vi "Graph Data.vi"(8 "error in (no error)":errorcluster, 10 "signal out":waveform(dbl), 11 "GUI_Graph in":refnum<class "GUI_Graph.lvclass">) -> (0 "error out":errorcluster, 3 "GUI_Graph out":refnum<class "GUI_Graph.lvclass">)   [LabVIEW 2020, in "GUI_Graph.lvlib" / "GUI_Graph.lvclass"]
uses:
  GUI_Graph.lvclass
  GUI_Graph.lvclass/GUI_Graph.ctl
  Loggin/Loggin Messages/Save Data Msg/Save Data Msg.lvclass/Save Data Msg.ctl
  <vilib>/ActorFramework/Message Enqueuer/Message Enqueuer.lvclass/Message Enqueuer.ctl
  <vilib>/ActorFramework/Message Enqueuer/Enqueue.vi
  Loggin/Loggin Messages/Save Data Msg/Save Data Msg.lvclass
  C:/Program Files/National Instruments/LabVIEW 2020/vi.lib/ActorFramework/Message/Message.lvclass
  <vilib>/ActorFramework/Message Priority Queue/Priority Enqueue.vi
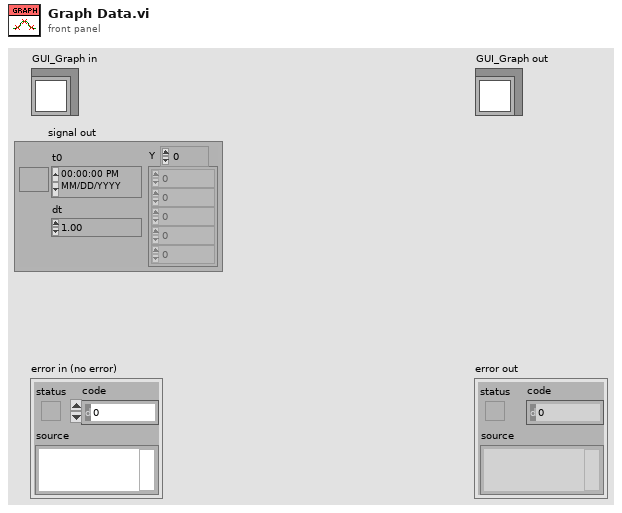
[diagram p1: front panel]
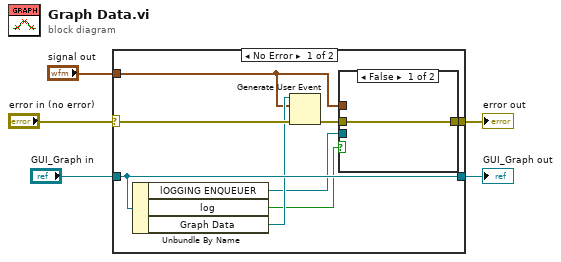
[diagram p0: block diagram]
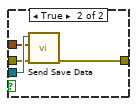
[diagram p2: hidden frame]
diagram:
  n1 = case shown="No Error" "error in (no error)" {
    selector: "error in (no error)" -> [w12 w20]
    tunnel: [w6 w20] -> w4
    tunnel: [w13 w19] -> w2
    tunnel: "GUI_Graph in" -> [w13 w19]
    tunnel: "signal out" -> [w8 _]
    frame No Error {
      n2 = Unbundle By Name(w13) -> ("lOGGING ENQUEUER"=w9:refnum<class "Message Enqueuer.lvclass">, "log"=w10:bool, "Graph Data"=w11:refnum<user-event>)
      n3 = Generate User Event(user event=w11, event data cluster=w8, error in=w12) -> (error out=w7:errorcluster)  [unwired: 1 in, 1 out]
      n4 = case shown="False" w10 {
        tunnel: w9 -> [_ w18]
        tunnel: w8 -> [_ w17]
        tunnel: w7 -> [w14 w16]
        tunnel: [w14 w15] -> w6
        frame False {
        }
        frame True {
          n5 = call "Send Save Data.vi"("error in (no error)"=w16, "signal out"=w17, "Message Enqueuer"=w18) -> ("error out"=w15:errorcluster)  [unwired: 7 in, 1 out]
        }
      }
    }
    frame Error {
    }
  }
  "error out" <- w4
  "GUI_Graph out" <- w2
